vi "Aotumation intergral.vi"() -> ()   [LabVIEW 2020]
uses:
  <vilib>/Instr/_visa.llb/VISA Configure Serial Port (Instr).vi
panel:
  in  "Tab Control":enum32{"Page 1"}(tab)
  in  "Motors VISA resource 2":refnum<visa-resource-name>="COM15"
  out "Total Image":dbl=10.0
  in  "Wavelength Filter VISA resource":refnum<visa-resource-name>="COM6"
  in  "Bandwidth":dbl=10.0
  in  "Shortest centroid":dbl=400.0
  in  "Sampling range":dbl=5.0
  in  "Longest centroid":dbl=700.0
  out "Wavelength Filter Currently State :":string
  in  "Step Angle (analyzer)":dbl=10.0 format="%#_13g"
  out "?":dbl(knob) scale=0.0..360.0
  out "Currently Angle : (Analyzer)":string
  in  "iXon exposure time (sec)":dbl=0.15
  in  "½Ð¤Å«ö¥ª¤W¨¤ªº°±¤îµ{¦¡":bool
  in  "Stop":bool
  in  "?":bool
  out "B_Degree":dbl
  out "A_Degree":dbl
  in  "A incre. degree":dbl=1.0
  in  "B incre.  degree":dbl=1.0
  in  "B(Detector) incremental":bool
  in  "A(Laser) incremental":bool
  in  "A STOP":bool
  in  "B STOP":bool
  in  "A set 0":bool
  in  "B set 0":bool
  in  "Find Circle central mode\nStart with A=25 ,B= -25\nStop: during the homing time":bool
  in  "Motors VISA resource":refnum<visa-resource-name>="COM8"
  out "?":dbl(slide) scale=400.0..700.0
  out "Goniometer":cluster{"Numeric 3":dbl, "Numeric 3":dbl}(knob)={"Numeric 3"=0.0, "Numeric 3"=113.9092127165585} scale=0.0..180.0
  out "Angle Of Incident":dbl
  out "Hours  2":dbl
  out "Minutes":dbl
  out "Seconds  2":dbl
  in  "B JOG":bool
  in  "A JOG":bool
  in  "A JOG  acc. set":bool
  in  "B JOG  acc. set":bool
  in  "AB STOP":bool
  in  "B acc. time(ms)":bool
  in  "A acc. time(ms)":bool
  in  "B velocity set":bool
  in  "A velocity set":bool
  in  "B velocity":dbl=600.0 format="%#_13g"
  in  "B acc. time":dbl=500.0 format="%#_13g"
  in  "A acc.time":dbl=500.0 format="%#_13g"
  in  "A velocity":dbl=600.0 format="%#_13g"
  in  "B JOG V value":dbl=600.0 format="%#_13g"
  in  "A JOG V value":dbl=600.0 format="%#_13g"
  # "Arm Setting\nA=Laser arm, B=Detector arm"
  # "Wavelength Filter Setting"
  # "Mortor Setting"
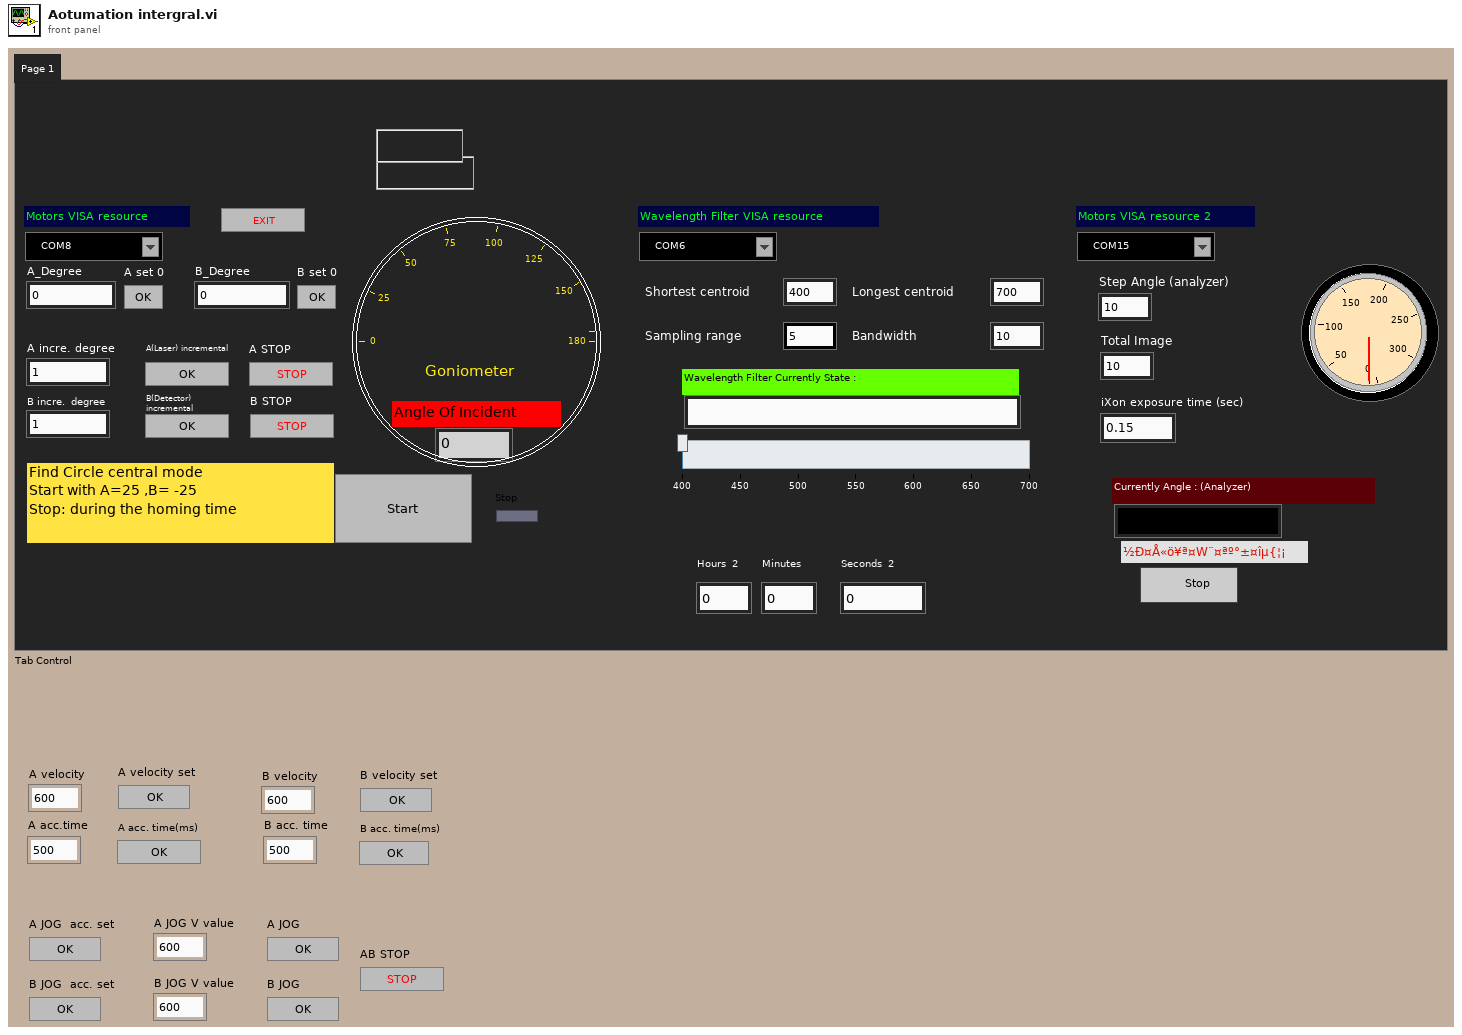
[diagram p1: front panel]
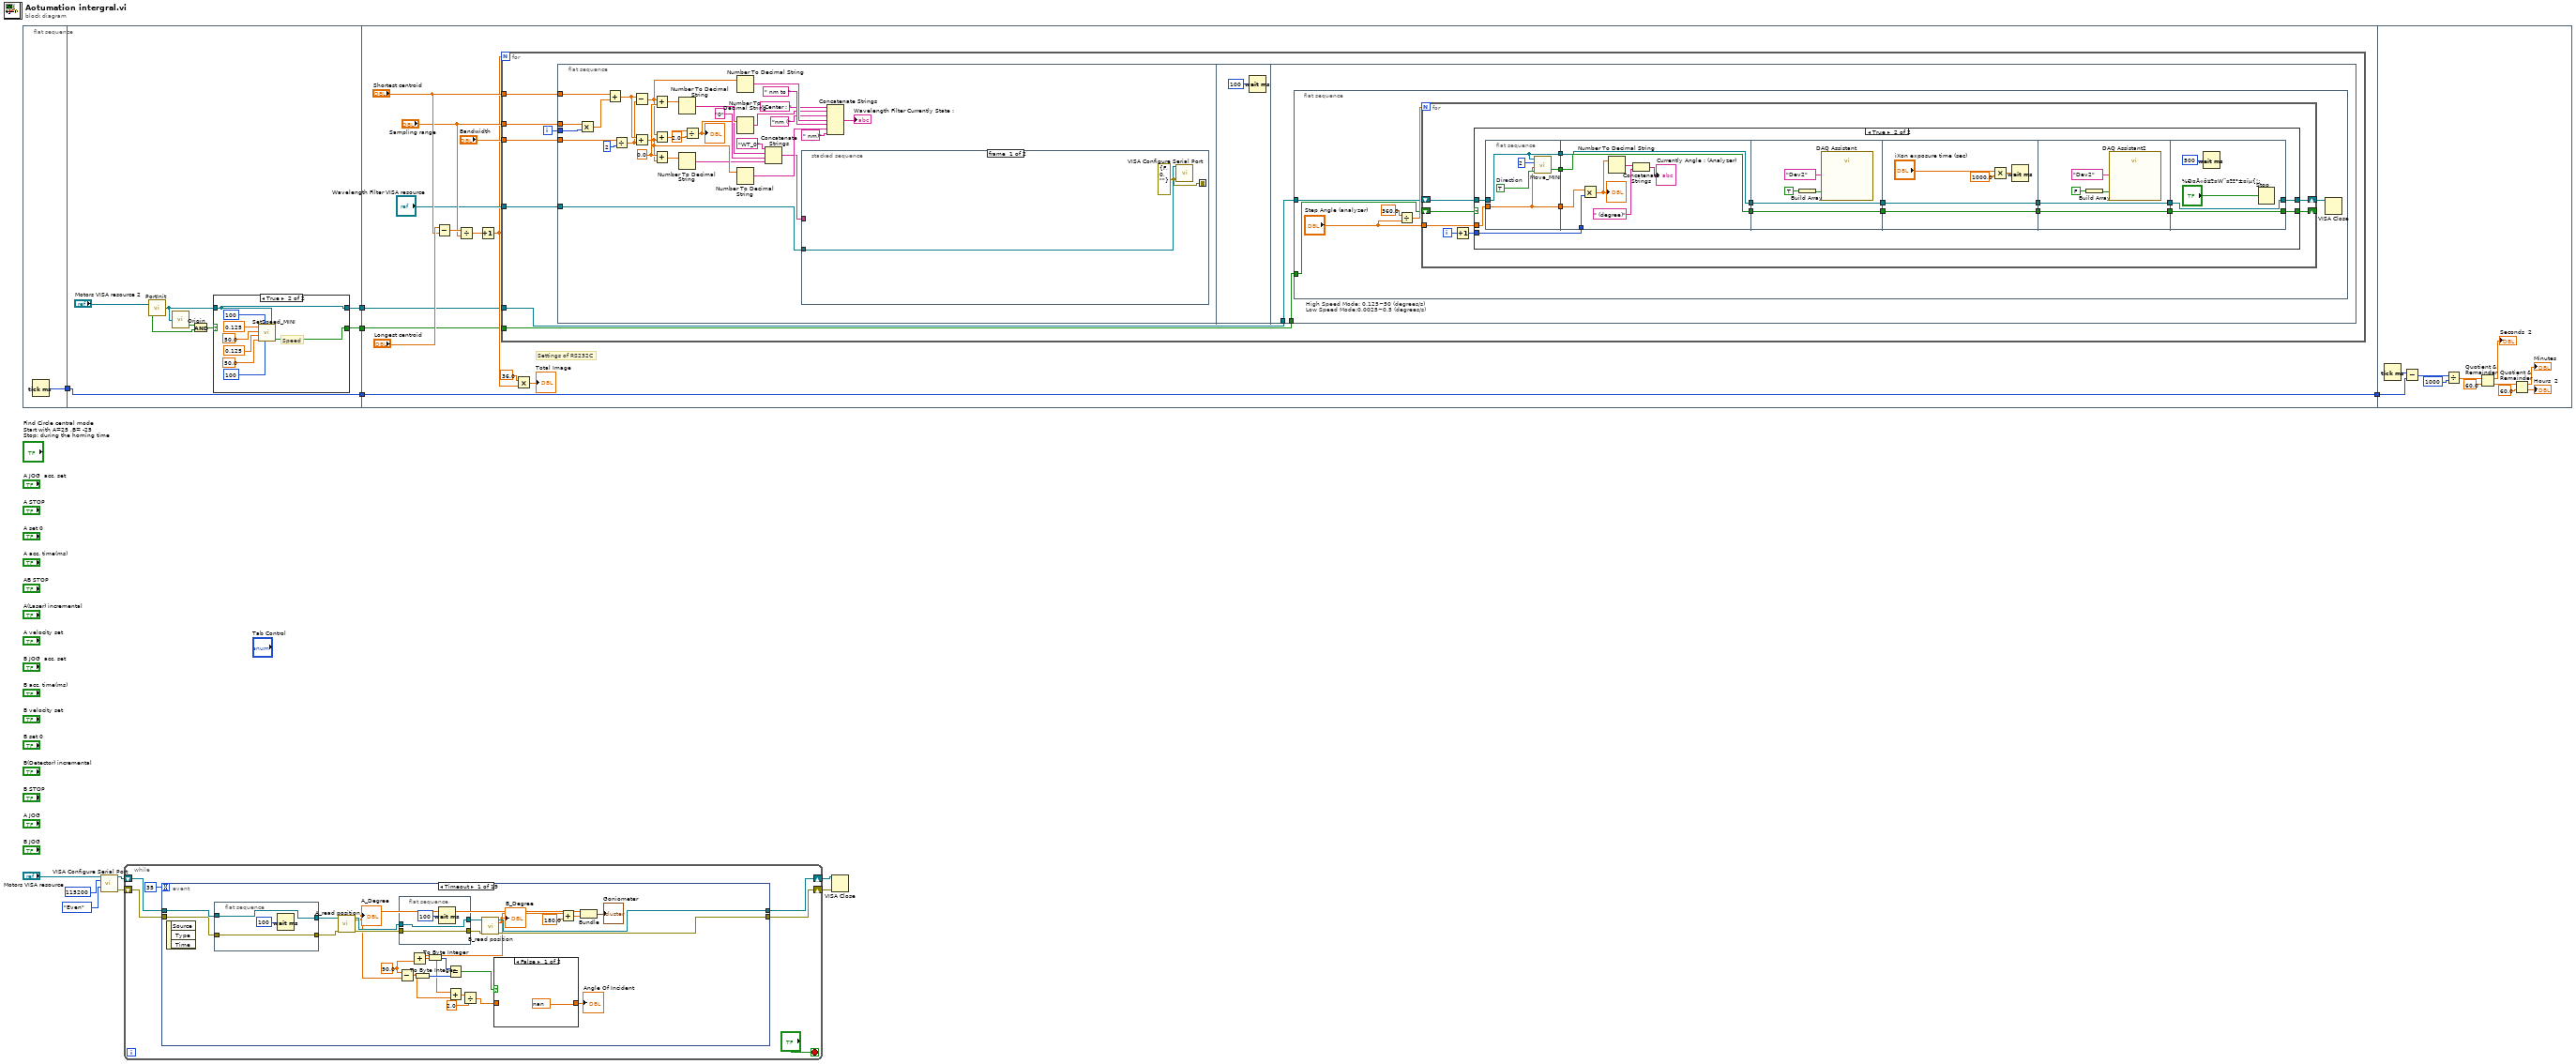
[diagram p0: block diagram]
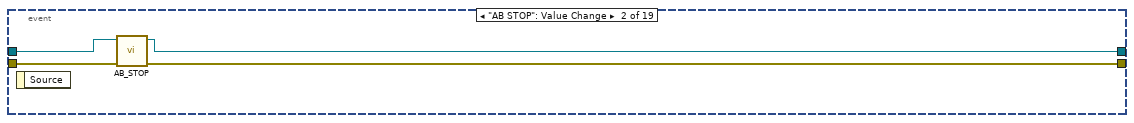
[diagram p3: hidden frame]
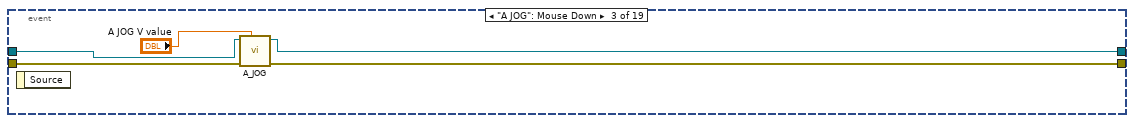
[diagram p4: hidden frame]
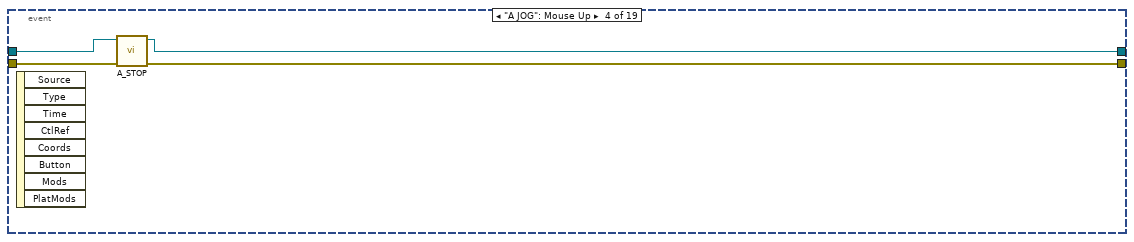
[diagram p5: hidden frame]
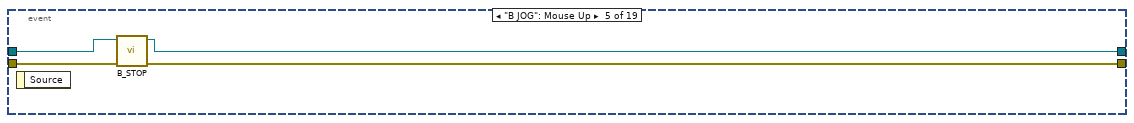
[diagram p6: hidden frame]
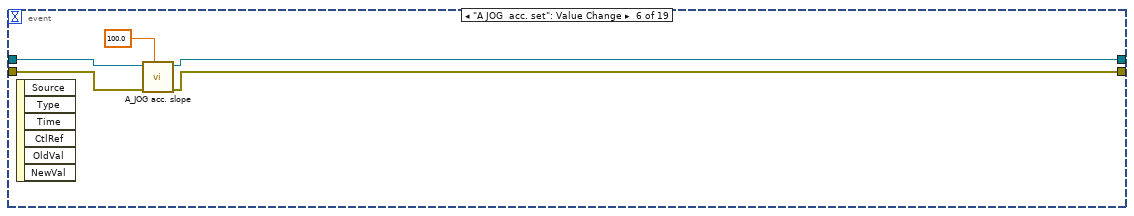
[diagram p7: hidden frame]
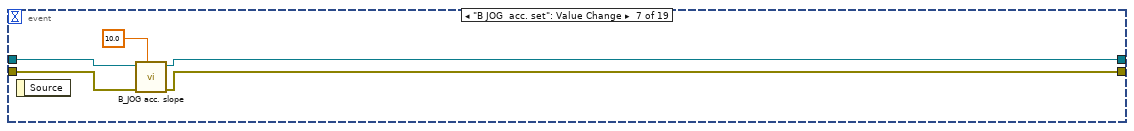
[diagram p8: hidden frame]
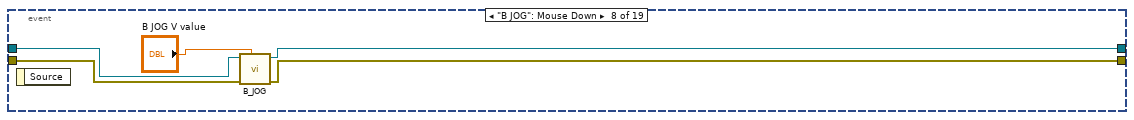
[diagram p9: hidden frame]
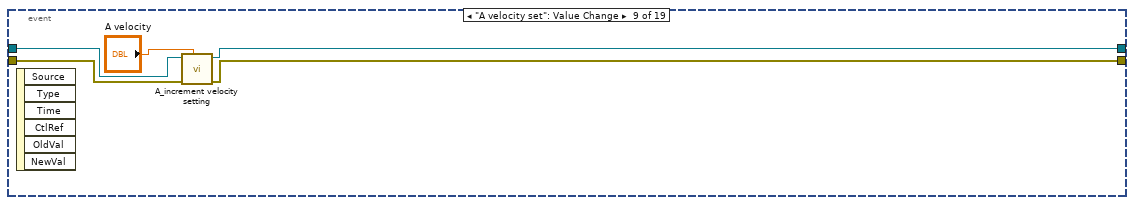
[diagram p10: hidden frame]
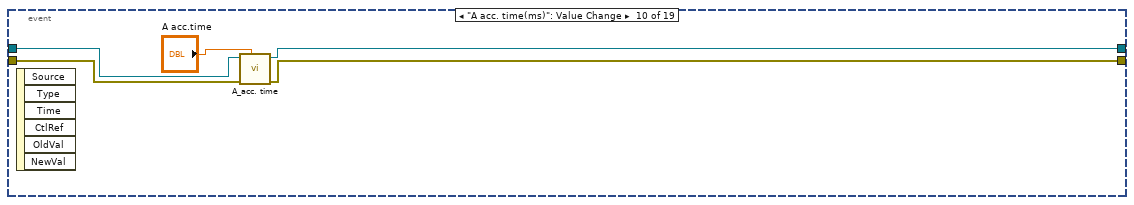
[diagram p11: hidden frame]
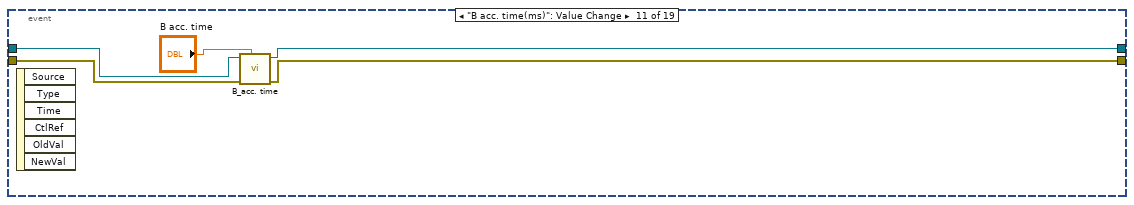
[diagram p12: hidden frame]
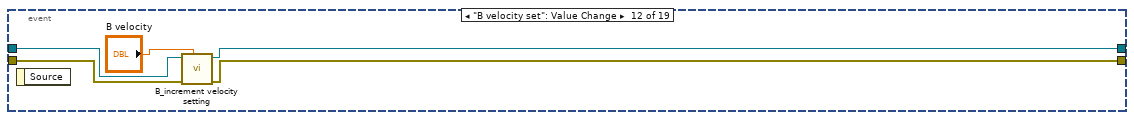
[diagram p13: hidden frame]
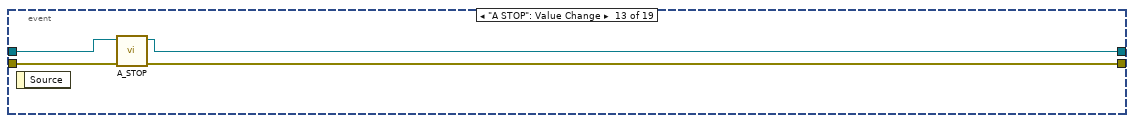
[diagram p14: hidden frame]
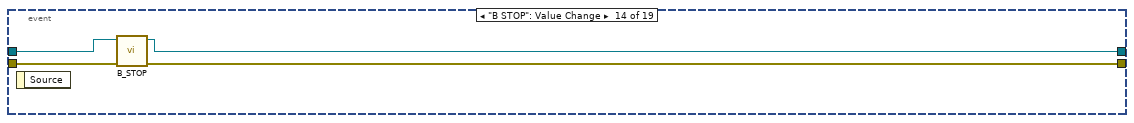
[diagram p15: hidden frame]
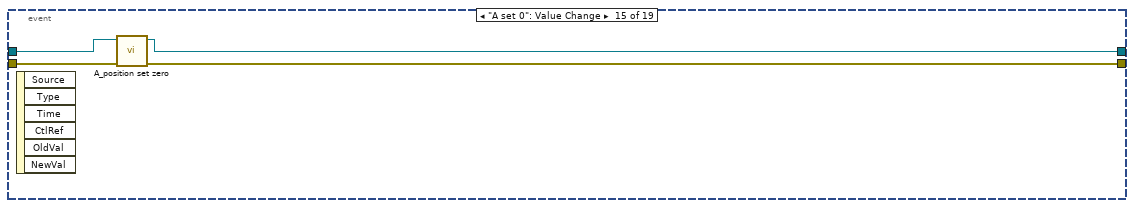
[diagram p16: hidden frame]
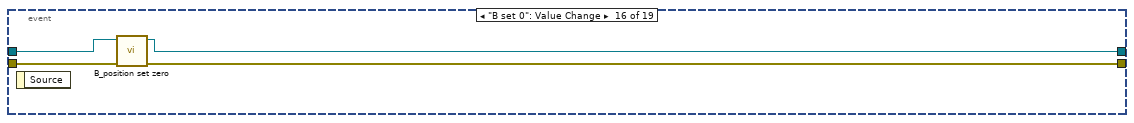
[diagram p17: hidden frame]
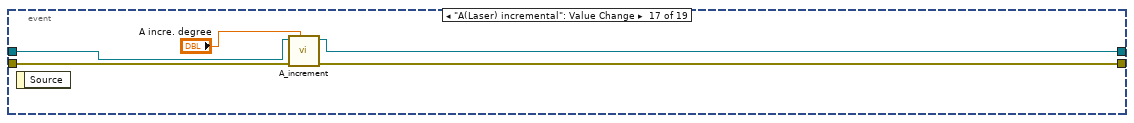
[diagram p18: hidden frame]
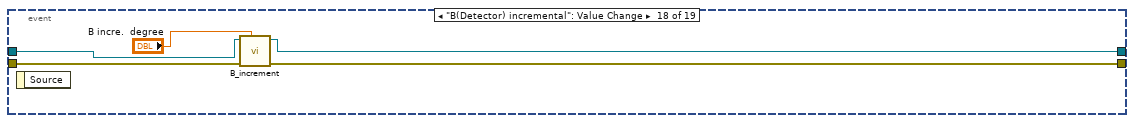
[diagram p19: hidden frame]
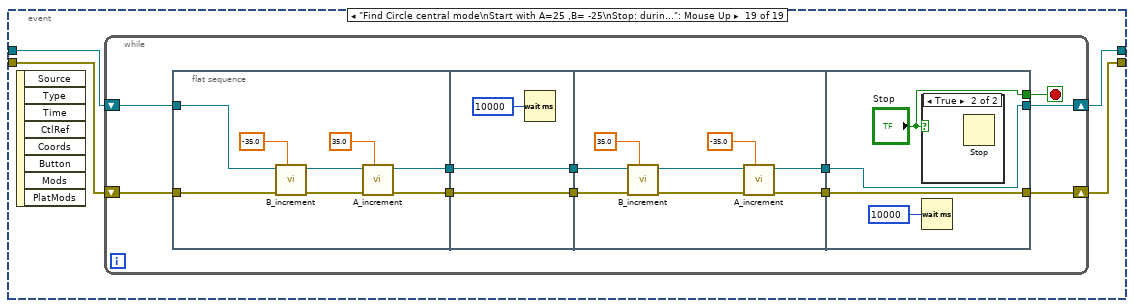
[diagram p20: hidden frame]
diagram:
  n1 = flat-sequence {
    tunnel: [w13] -> w12
    tunnel: w12 -> [w21]
    tunnel: [w21] -> w11
    tunnel: [w15] -> w10
    tunnel: [w14] -> w9
    tunnel: [w37] -> w8
    tunnel: w11 -> [w37]
    tunnel: w10 -> [w33]
    tunnel: w9 -> [w32]
    tunnel: w8 -> [w184]
    frame #0 {
      n2 = Tick Count (ms)() -> (millisecond timer value=w13:u32)
    }
    frame #1 {
      n3 = call "PortInit.vi"("VISAリソース名"="Motors VISA resource 2") -> ("VISA resource name out"=w16:refnum<visa-resource-name>, "Done"=w19:bool)
      n4 = call "Origin.vi"("VISAリソース名"=w16) -> ("OK Done"=w20:bool)  [unwired: 2 out]
      n5 = Compound Arithmetic op=AND(w20, w19) -> (w17:bool)
      n6 = case shown="True" w17 {
        tunnel: [w23 w31] -> w15
        tunnel: w16 -> [w22 w24]
        tunnel: [w22 w24] -> w14
        frame False {
          w23 = FALSE  # Direction
        }
        frame True {
          # "Speed"
          n7 = call "SetSpeed_MINI.vi"("VISAリソース名"=w24, "Acceleration Time2(ms)"=u32 100 ("Acceleration Time 2"), "Acceleration Time1(ms)"=u32 100 ("Acceleration Time 1"), "High Speed2(degrees/s)"=50.0 ("Polarizer Speed"), "Low Speed2(degrees/s)"=0.125 ("Axis 2 Low Speed"), "High Speed1(degrees/s)"=50.0 ("Analyzer Speed"), "Low Speed1(degrees/s)"=0.125 ("Axis 1 Low Speed")) -> ("OK Done"=w31:bool)  [unwired: 2 out]
        }
      }
    }
    frame #2 {
      # "Settings of RS232C"
      n8 = Subtract(x="Longest centroid", y="Shortest centroid") -> (x-y=w43:dbl)
      n9 = Divide(x=w43, y="Sampling range") -> (x/y=w39:dbl)
      n10 = Increment(x=w39) -> (x+1=w35:dbl)
      n11 = for {
        N: w35 -> [_]
        tunnel: "Shortest centroid" -> [w50]
        tunnel: "Sampling range" -> [w49]
        tunnel: "Bandwidth" -> [w48]
        tunnel: "Wavelength Filter VISA resource" -> [w47]
        tunnel: w33 -> [w46]
        tunnel: w32 -> [w45]
        i -> [w51]
        n12 = flat-sequence {
          tunnel: w51 -> [w67]
          tunnel: w50 -> [w73]
          tunnel: w49 -> [w72]
          tunnel: w48 -> [w71]
          tunnel: w47 -> [w59]
          tunnel: w45 -> [w120]
          tunnel: w46 -> [w119]
          frame #0 {
            w58 = 0.0 ("y")
            n13 = Multiply(x=w72, y=w67) -> (x*y=w70:dbl)
            n14 = Add(x=w73, y=w70) -> (x+y=w69:dbl)
            n15 = Divide(x=w71, y=2) -> (x/y=w68:dbl)
            n16 = Subtract(x=w69, y=w68) -> (x-y=w57:dbl)
            n17 = Add(x=w69, y=w68) -> (x+y=w54:dbl)
            n18 = Add(x=w57, y=w58) -> (x+y=w56:dbl)
            n19 = Add(x=w57, y=w54) -> (x+y=w65:dbl)
            n20 = Add(x=w58, y=w54) -> (x+y=w53:dbl)
            n21 = Number To Decimal String(number=w56) -> (decimal integer string=w55:string)  [unwired: 1 in]
            n22 = Number To Decimal String(number=w53) -> (decimal integer string=w52:string)  [unwired: 1 in]
            n23 = Divide(x=w65, y=2.0) -> (x/y=w63:dbl)
            "?" <- w63
            n24 = Number To Decimal String(number=w57) -> (decimal integer string=w76:string)  [unwired: 1 in]
            n25 = Number To Decimal String(number=w63) -> (decimal integer string=w62:string)  [unwired: 1 in]
            n26 = Number To Decimal String(number=w54) -> (decimal integer string=w75:string)  [unwired: 1 in]
            n27 = Concatenate Strings("WT_0", w55, "0", w52) -> (w74:string)
            n28 = stacked-sequence {
              seq-local: [w83 _] -> [_ w86]
              tunnel: w59 -> [w82 w85]
              tunnel: w74 -> [_ w84]
              frame #0 {
                w83 = errorcluster {"status"=FALSE, "code"=0, "source"=""} ("Error In (no error)")
                n29 = call-poly "VISA Configure Serial Port"("VISA resource name"=w82, "error in (no error)"=w83) -> ()  [unwired: 12 in, 2 out]
              }
              frame #1 {
                n30 = stacked-sequence {
                  seq-local: [w89 _] -> [_ w103]
                  seq-local: [w88 _] -> [_ w102]
                  tunnel: w85 -> [w91 _]
                  tunnel: w86 -> [w90 _]
                  tunnel: w84 -> [w87 _]
                  frame #0 {
                    n31 = case shown="No Error" w90 {
                      selector: w90 -> [w98 w100]
                      tunnel: w91 -> [w99 w101]
                      tunnel: [w97 w100] -> w88
                      tunnel: [w96 w101] -> w89
                      tunnel: w87 -> [w92 _]
                      frame No Error {
                        n32 = Concatenate Strings(w92, "\r", "\n") -> (w95:string)
                        n33 = VISA Write(VISA resource name=w99, write buffer=w95, error in (no error)=w98) -> (VISA resource name out=w96:refnum<visa-resource-name>, error out=w97:errorcluster)  [unwired: 1 out]
                      }
                      frame Error {
                      }
                    }
                  }
                  frame #1 {
                    n34 = case shown="No Error" w102 {
                      selector: w102 -> [w109 w117]
                      tunnel: [w106 w117] -> w104
                      tunnel: w103 -> [w110 w116]
                      tunnel: [w107 w116] -> w105
                      frame No Error {
                        # "Error False: Read\nWith Timeout Executed"
                        n35 = Multiply(x=5.0 ("Timeout Limit (s)(10)"), y=1000) -> (x*y=w111:dbl)
                        n36 = property class="Instr"(reference=w110, error in=w109, "General Settings:Timeout Value"=w111) -> (reference out=w115:refnum<visa-resource-name>, error out=w114:errorcluster)
                        n37 = VISA Read(VISA resource name=w115, byte count=30 ("Bytes To Read (30)"), error in (no error)=w114) -> (VISA resource name out=w107:refnum<visa-resource-name>, error out=w106:errorcluster)  [unwired: 2 out]
                      }
                      frame Error {
                      }
                    }
                    n38 = VISA Close(VISA resource name=w105, error in (no error)=w104) -> ()  [unwired: 1 out]
                  }
                }
              }
            }
            n39 = Concatenate Strings("Center : " ("string"), w62, "nm (" ("string"), w76, " nm to ", w75, " nm)" ("string")) -> (→"Wavelength Filter Currently State :":string)
          }
          frame #1 {
            n40 = Wait (ms)(milliseconds to wait=u32 100) -> ()  [unwired: 1 out]
          }
          frame #2 {
            # "High Speed Mode: 0.125~50 (degrees/s)\nLow Speed Mode:0.0025~0.5 (degrees/s)"
            n41 = flat-sequence {
              tunnel: w120 -> [w122]
              tunnel: w119 -> [w121]
              frame #0 {
                n42 = Divide(x=360.0 ("y"), y="Step Angle (analyzer)") -> (x/y=w123:dbl)
                n43 = for {
                  N: w123 -> [_]
                  shift-right: [w128] -> _
                  shift-left: w121 -> [w133]
                  shift-right: [w129] -> w126
                  shift-left: w122 -> [w132]
                  tunnel: "Step Angle (analyzer)" -> [w131]
                  i -> [w130]
                  n44 = Increment(x=w130) -> (x+1=w127:i32)
                  n45 = case shown="True" w133 {
                    selector: w133 -> [w135 _]
                    tunnel: [w135 w143] -> w128
                    tunnel: w132 -> [w134 w151]
                    tunnel: [w134 w137] -> w129
                    tunnel: w127 -> [_ w149]
                    tunnel: w131 -> [_ w148]
                    frame False {
                    }
                    frame True {
                      n46 = flat-sequence {
                        tunnel: w148 -> [w152]
                        tunnel: w151 -> [w153]
                        tunnel: [w156] -> w150
                        tunnel: [w153] -> w141
                        tunnel: [w152] -> w136
                        tunnel: w150 -> [w164]
                        tunnel: w149 -> [w160]
                        tunnel: [w164] -> w147
                        tunnel: [w158] -> w142
                        tunnel: w141 -> [w158]
                        tunnel: w136 -> [w157]
                        tunnel: w147 -> [w169]
                        tunnel: [w169] -> w146
                        tunnel: w142 -> [w168]
                        tunnel: [w168] -> w140
                        tunnel: w146 -> [w174]
                        tunnel: [w174] -> w145
                        tunnel: w140 -> [w170]
                        tunnel: [w170] -> w139
                        tunnel: w145 -> [w179]
                        tunnel: [w179] -> w144
                        tunnel: w139 -> [w177]
                        tunnel: [w177] -> w138
                        tunnel: [w183] -> w143
                        tunnel: w144 -> [w183]
                        tunnel: w138 -> [w181]
                        tunnel: [w181] -> w137
                        frame #0 {
                          w155 = TRUE  # Direction
                          n47 = call "Move_MINI.vi"("Direction"=w155, "Step Angle(degree)"=w152, "Axis Number"=2 ("AxisNumber"), "VISAリソース名"=w153) -> ("OK Done"=w156:bool)  [unwired: 1 in]
                        }
                        frame #1 {
                          n48 = Multiply(x=w157, y=w160) -> (x*y=w159:dbl)
                          "?" <- w159
                          n49 = Number To Decimal String(number=w159) -> (decimal integer string=w163:string)  [unwired: 1 in]
                          n50 = Concatenate Strings(w163, " (degree)" ("string")) -> (→"Currently Angle : (Analyzer)":string)
                        }
                        frame #2 {
                          n51 = Build Array(TRUE) -> (w165:bool[])
                          n52 = call "DAQ Assistant"("data"=w165, "device name"=tag "Dev2") -> ()  [unwired: 16 in, 2 out]
                        }
                        frame #3 {
                          n53 = Multiply(x="iXon exposure time (sec)", y=1000.0) -> (x*y=w172:dbl)
                          n54 = Wait (ms)(milliseconds to wait=w172) -> ()  [unwired: 1 out]
                        }
                        frame #4 {
                          n55 = Build Array(FALSE) -> (w175:bool[])
                          n56 = call "DAQ Assistant2"("data"=w175, "device name"=tag "Dev2") -> ()  [unwired: 16 in, 2 out]
                        }
                        frame #5 {
                          n57 = Wait (ms)(milliseconds to wait=u32 500) -> ()  [unwired: 1 out]
                          n58 = Stop(stop? (T)="½Ð¤Å«ö¥ª¤W¨¤ªº°±¤îµ{¦¡") -> ()
                        }
                      }
                    }
                  }
                }
                n59 = VISA Close(VISA resource name=w126) -> ()  [unwired: 1 in, 1 out]
              }
            }
          }
        }
      }
      n60 = Multiply(x=36.0, y=w35) -> (x*y=→"Total Image":dbl)
    }
    frame #3 {
      n61 = Tick Count (ms)() -> (millisecond timer value=w191:u32)
      n62 = Subtract(x=w191, y=w184) -> (x-y=w192:u32)
      n63 = Divide(x=w192, y=u32 1000) -> (x/y=w193:dbl)
      n64 = Quotient & Remainder(x=w193, y=60.0) -> (x-y*floor(x/y)=→"Seconds  2":dbl, floor(x/y)=w194:dbl)
      n65 = Quotient & Remainder(x=w194, y=60.0) -> (x-y*floor(x/y)=→"Minutes":dbl, floor(x/y)=→"Hours  2":dbl)
    }
  }
  n66 = call-poly "VISA Configure Serial Port"("VISA resource name"="Motors VISA resource", "baud rate (9600)"=u32 115200, "parity (0:none)"=enum16{"None", "Odd", "Even", "Mark", "Space"}."Even") -> ("VISA resource name out"=w5:refnum<visa-resource-name>, "error out"=w4:errorcluster)  [unwired: 11 in]
  n67 = while {
    shift-right: [w197] -> w3
    shift-left: w5 -> [w199]
    shift-right: [w196] -> w2
    shift-left: w4 -> [w198]
    stop <- "?" stop-if-true
    n68 = event shown="[0] Timeout" {
      selector: _ -> [_ _ _ _ _ _ _ _ _ _ _ _ _ _ _ _ _ _ _]
      dyn-events: _ -> [_ _ _ _ _ _ _ _ _ _ _ _ _ _ _ _ _ _ _]
      timeout: 35 -> [_ _ _ _ _ _ _ _ _ _ _ _ _ _ _ _ _ _ _]
      tunnel: w199 -> [w221 w237 w242 w246 w250 w255 w260 w265 w270 w275 w280 w285 w289 w293 w297 w301 w306 w311 w314]
      tunnel: w198 -> [w220 w236 w241 w245 w249 w254 w259 w264 w269 w274 w279 w284 w288 w292 w296 w300 w305 w310 w315]
      tunnel: [w223 w235 w240 w244 w248 w253 w258 w263 w267 w273 w278 w283 w287 w291 w295 w299 w304 w309 w313] -> w197
      tunnel: [w222 w234 w239 w243 w247 w252 w257 w262 w266 w272 w277 w282 w286 w290 w294 w298 w303 w308 w312] -> w196
      event Timeout {
        w211 = 90.0 ("x")
        n69 = event-data() -> ()  [unwired: 1 in, 3 out]
        n70 = flat-sequence {
          tunnel: [w229] -> w219
          tunnel: w221 -> [w229]
          tunnel: w220 -> [w228]
          tunnel: [w228] -> w216
          frame #0 {
            n71 = Wait (ms)(milliseconds to wait=u32 100) -> ()  [unwired: 1 out]
          }
        }
        n72 = call "A_read position.vi"("VISA resource name"=w219, "error in (no error)"=w216) -> ("A_Degree"=w212:dbl, "VISA resource name out"=w218:refnum<visa-resource-name>, "error out"=w217:errorcluster)  [unwired: 5 in]
        "A_Degree" <- w212
        n73 = flat-sequence {
          tunnel: [w232] -> w225
          tunnel: w218 -> [w232]
          tunnel: w217 -> [w231]
          tunnel: [w231] -> w224
          frame #0 {
            n74 = Wait (ms)(milliseconds to wait=u32 100) -> ()  [unwired: 1 out]
          }
        }
        n75 = Subtract(x=w211, y=w212) -> (x-y=w205:dbl)
        n76 = To Byte Integer(number=w205) -> (8bit integer=w209:i8)
        n77 = call "B_read position.vi"("error in (no error)"=w224, "VISA resource name"=w225) -> ("error out"=w222:errorcluster, "VISA resource name out"=w223:refnum<visa-resource-name>, "B_Degree"=w210:dbl)  [unwired: 7 in]
        "B_Degree" <- w210
        n78 = Add(x=w210, y=w211) -> (x+y=w206:dbl)
        n79 = To Byte Integer(number=w206) -> (8bit integer=w208:i8)
        n80 = Equal?(x=w208, y=w209) -> (x = y?=w207:bool)
        n81 = Add(x=w206, y=w205) -> (x+y=w204:dbl)
        n82 = Divide(x=w204, y=2.0) -> (x/y=w202:dbl)
        n83 = case shown="False" w207 {
          tunnel: w202 -> [_ w227]
          tunnel: [nan w227] -> w201
          frame False {
          }
          frame True {
          }
        }
        "Angle Of Incident" <- w201
        n84 = Add(x=w210, y=180.0) -> (x+y=w213:dbl)
        n85 = Bundle("A_Degree"=w212, w213) -> (→"Goniometer":cluster{"A_Degree":dbl, dbl})  [unwired: 1 in]
      }
      event "AB STOP": Value Change {
        n86 = event-data() -> ()  [unwired: 1 in, 1 out]
        n87 = call "AB_STOP.vi"("VISA resource name"=w237, "error in (no error)"=w236) -> ("VISA resource name out"=w235:refnum<visa-resource-name>, "error out"=w234:errorcluster)  [unwired: 7 in]
      }
      event "A JOG": Mouse Down {
        n88 = event-data() -> ()  [unwired: 1 in, 1 out]
        n89 = call "A_JOG.vi"("Degree per min"="A JOG V value", "error in (no error)"=w241, "VISA resource name"=w242) -> ("error out"=w239:errorcluster, "VISA resource name out"=w240:refnum<visa-resource-name>)  [unwired: 7 in]
      }
      event "A JOG": Mouse Up {
        n90 = event-data() -> ()  [unwired: 1 in, 8 out]
        n91 = call "A_STOP.vi"("VISA resource name"=w246, "error in (no error)"=w245) -> ("VISA resource name out"=w244:refnum<visa-resource-name>, "error out"=w243:errorcluster)  [unwired: 7 in]
      }
      event "B JOG": Mouse Up {
        n92 = event-data() -> ()  [unwired: 1 in, 1 out]
        n93 = call "B_STOP.vi"("VISA resource name"=w250, "error in (no error)"=w249) -> ("VISA resource name out"=w248:refnum<visa-resource-name>, "error out"=w247:errorcluster)  [unwired: 7 in]
      }
      event "A JOG  acc. set": Value Change {
        n94 = event-data() -> ()  [unwired: 1 in, 6 out]
        n95 = call "A_JOG acc. slope.vi"("(Degree/min)/s"=100.0 ("A JOG acc.set"), "error in (no error)"=w254, "VISA resource name"=w255) -> ("error out"=w252:errorcluster, "VISA resource name out"=w253:refnum<visa-resource-name>)  [unwired: 5 in]
      }
      event "B JOG  acc. set": Value Change {
        n96 = event-data() -> ()  [unwired: 1 in, 1 out]
        n97 = call "B_JOG acc. slope.vi"("(Degree/min)/s"=10.0 ("B JOG acc.set"), "error in (no error)"=w259, "VISA resource name"=w260) -> ("error out"=w257:errorcluster, "VISA resource name out"=w258:refnum<visa-resource-name>)  [unwired: 5 in]
      }
      event "B JOG": Mouse Down {
        n98 = event-data() -> ()  [unwired: 1 in, 1 out]
        n99 = call "B_JOG.vi"("Degree per min"="B JOG V value", "error in (no error)"=w264, "VISA resource name"=w265) -> ("error out"=w262:errorcluster, "VISA resource name out"=w263:refnum<visa-resource-name>)  [unwired: 7 in]
      }
      event "A velocity set": Value Change {
        n100 = event-data() -> ()  [unwired: 1 in, 6 out]
        n101 = call "A_increment velocity setting.vi"("Degree per min"="A velocity", "error in (no error)"=w269, "VISA resource name"=w270) -> ("error out"=w266:errorcluster, "VISA resource name out"=w267:refnum<visa-resource-name>)  [unwired: 5 in]
      }
      event "A acc. time(ms)": Value Change {
        n102 = event-data() -> ()  [unwired: 1 in, 6 out]
        n103 = call "A_acc. time.vi"("ms"="A acc.time", "error in (no error)"=w274, "VISA resource name"=w275) -> ("error out"=w272:errorcluster, "VISA resource name out"=w273:refnum<visa-resource-name>)  [unwired: 7 in]
      }
      event "B acc. time(ms)": Value Change {
        n104 = event-data() -> ()  [unwired: 1 in, 6 out]
        n105 = call "B_acc. time.vi"("Degree per second"="B acc. time", "error in (no error)"=w279, "VISA resource name"=w280) -> ("error out"=w277:errorcluster, "VISA resource name out"=w278:refnum<visa-resource-name>)  [unwired: 7 in]
      }
      event "B velocity set": Value Change {
        n106 = event-data() -> ()  [unwired: 1 in, 1 out]
        n107 = call "B_increment velocity setting.vi"("Degree per min"="B velocity", "error in (no error)"=w284, "VISA resource name"=w285) -> ("error out"=w282:errorcluster, "VISA resource name out"=w283:refnum<visa-resource-name>)  [unwired: 5 in]
      }
      event "A STOP": Value Change {
        n108 = event-data() -> ()  [unwired: 1 in, 1 out]
        n109 = call "A_STOP.vi"("VISA resource name"=w289, "error in (no error)"=w288) -> ("VISA resource name out"=w287:refnum<visa-resource-name>, "error out"=w286:errorcluster)  [unwired: 7 in]
      }
      event "B STOP": Value Change {
        n110 = event-data() -> ()  [unwired: 1 in, 1 out]
        n111 = call "B_STOP.vi"("VISA resource name"=w293, "error in (no error)"=w292) -> ("VISA resource name out"=w291:refnum<visa-resource-name>, "error out"=w290:errorcluster)  [unwired: 7 in]
      }
      event "A set 0": Value Change {
        n112 = event-data() -> ()  [unwired: 1 in, 6 out]
        n113 = call "A_position set zero.vi"("error in (no error)"=w296, "VISA resource name"=w297) -> ("error out"=w294:errorcluster, "VISA resource name out"=w295:refnum<visa-resource-name>)  [unwired: 8 in]
      }
      event "B set 0": Value Change {
        n114 = event-data() -> ()  [unwired: 1 in, 1 out]
        n115 = call "B_position set zero.vi"("error in (no error)"=w300, "VISA resource name"=w301) -> ("error out"=w298:errorcluster, "VISA resource name out"=w299:refnum<visa-resource-name>)  [unwired: 8 in]
      }
      event "A(Laser) incremental": Value Change {
        n116 = event-data() -> ()  [unwired: 1 in, 1 out]
        n117 = call "A_increment.vi"("Degree"="A incre. degree", "error in (no error)"=w305, "VISA resource name 4"=w306) -> ("error out"=w303:errorcluster, "VISA resource name out"=w304:refnum<visa-resource-name>)  [unwired: 7 in]
      }
      event "B(Detector) incremental": Value Change {
        n118 = event-data() -> ()  [unwired: 1 in, 1 out]
        n119 = call "B_increment.vi"("Degree"="B incre.  degree", "error in (no error)"=w310, "VISA resource name 4"=w311) -> ("error out"=w308:errorcluster, "VISA resource name out"=w309:refnum<visa-resource-name>)  [unwired: 7 in]
      }
      event "Find Circle central mode\nStart with A=25 ,B= -25\nStop: during the homing time": Mouse Up {
        n120 = event-data() -> ()  [unwired: 1 in, 8 out]
        n121 = while {
          shift-right: [w323] -> w312
          shift-left: w315 -> [w326]
          shift-right: [w324] -> w313
          shift-left: w314 -> [w325]
          stop <- w316 stop-if-true
          n122 = flat-sequence {
            tunnel: w326 -> [w332]
            tunnel: w325 -> [w331]
            tunnel: [w328] -> w320
            tunnel: [w327] -> w318
            tunnel: w320 -> [w337]
            tunnel: [w337] -> w319
            tunnel: w318 -> [w336]
            tunnel: [w336] -> w317
            tunnel: w319 -> [w341]
            tunnel: w317 -> [w340]
            tunnel: [w339] -> w322
            tunnel: [w338] -> w321
            tunnel: [w348] -> w323
            tunnel: [w349] -> w324
            tunnel: w322 -> [w349]
            tunnel: w321 -> [w348]
            tunnel: ["Stop"] -> w316
            frame #0 {
              n123 = call "B_increment.vi"("Degree"=-35.0 ("B incre.  degree 2"), "error in (no error)"=w332, "VISA resource name 4"=w331) -> ("error out"=w329:errorcluster, "VISA resource name out"=w334:refnum<visa-resource-name>)  [unwired: 7 in]
              n124 = call "A_increment.vi"("Degree"=35.0 ("A incre. degree  2"), "error in (no error)"=w329, "VISA resource name 4"=w334) -> ("error out"=w327:errorcluster, "VISA resource name out"=w328:refnum<visa-resource-name>)  [unwired: 7 in]
            }
            frame #1 {
              n125 = Wait (ms)(milliseconds to wait=u32 10000) -> ()  [unwired: 1 out]
            }
            frame #2 {
              n126 = call "B_increment.vi"("Degree"=35.0 ("B incre.  degree 2"), "error in (no error)"=w340, "VISA resource name 4"=w341) -> ("error out"=w345:errorcluster, "VISA resource name out"=w344:refnum<visa-resource-name>)  [unwired: 7 in]
              n127 = call "A_increment.vi"("Degree"=-35.0 ("A incre. degree  2"), "error in (no error)"=w345, "VISA resource name 4"=w344) -> ("error out"=w338:errorcluster, "VISA resource name out"=w339:refnum<visa-resource-name>)  [unwired: 7 in]
            }
            frame #3 {
              n128 = case shown="True" "Stop" {
                frame False {
                }
                frame True {
                  n129 = Stop() -> ()  [unwired: 1 in]
                }
              }
              n130 = Wait (ms)(milliseconds to wait=u32 10000) -> ()  [unwired: 1 out]
            }
          }
        }
      }
    }
  }
  n131 = VISA Close(VISA resource name=w3, error in (no error)=w2) -> ()  [unwired: 1 out]
